vi "Initialize Core.vi"(8 "error in (no error)":errorcluster, 10 "Parameters":refnum<class "Abstract Init Parameters.lvclass">, 11 "Abstract Log Consumer in":refnum<class "Abstract Log Consumer.lvclass">) -> (0 "error out":errorcluster, 3 "Abstract Log Consumer out":refnum<class "Abstract Log Consumer.lvclass">)   [LabVIEW 2020]
uses:
  Abstract Log Consumer.lvclass
  Parameters/Abstract Init Parameters/Abstract Init Parameters.lvclass
  Consumer/Abstract Consumer/Abstract Consumer.lvclass
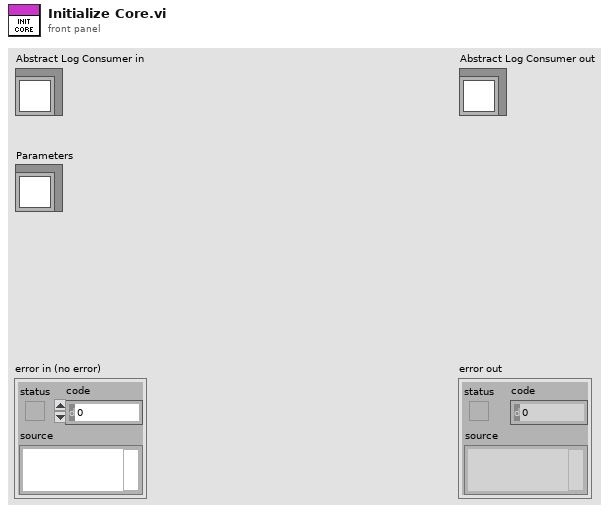
[diagram p1: front panel]
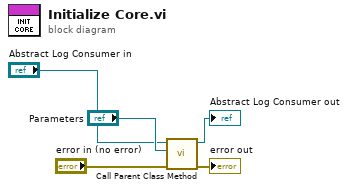
[diagram p0: block diagram]
diagram:
  n1 = call-parent "Call Parent Class Method"("error in (no error)"="error in (no error)", "Parameters"="Parameters", "Abstract Consumer in"="Abstract Log Consumer in") -> ("error out"=→"error out":errorcluster, "Abstract Consumer out"=→"Abstract Log Consumer out":refnum<class "Abstract Log Consumer.lvclass">)  [unwired: 7 in]
